vi "Tektronix ConfigOnly.vi"(5 "End Point":i32, 7 "Start Point":i32, 8 "error in (no error)":errorcluster, 9 "Waveform Width":u8(knob)=2 min=1 max=2 step=1 scale=0.0..2.0, 10 "# Average":u8(ring)=4 items=["128"=128, "64"=64, "16"=16, "4"=4], 11 "Tektronix (0::20:)":refnum<visa-resource-name>) -> (0 "error out":errorcluster, 1 "Waveform Parameters":string, 2 "Acquire Parameters":string, 3 "VISA resource name out":refnum<visa-resource-name>)   [LabVIEW 2018]
panel:
  out "concatenated string":string
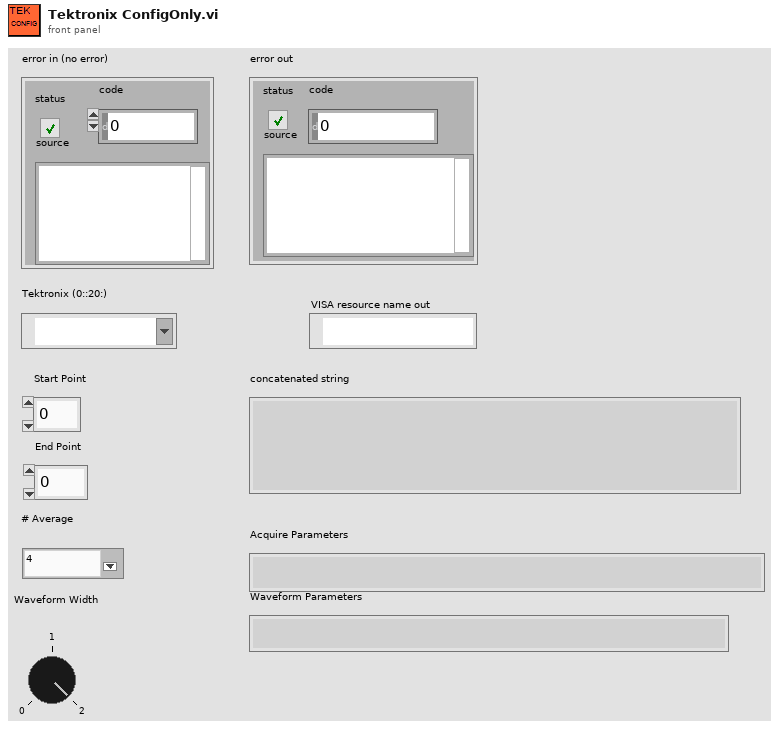
[diagram p1: front panel]
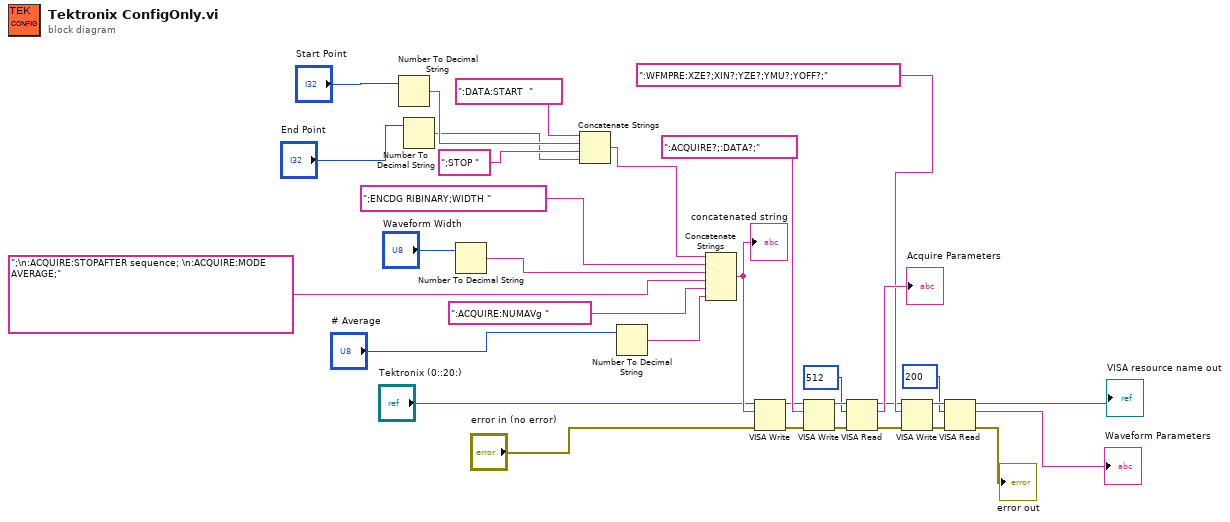
[diagram p0: block diagram]
diagram:
  n1 = Number To Decimal String(number="Start Point") -> (decimal integer string=w12:string)  [unwired: 1 in]
  n2 = Number To Decimal String(number="End Point") -> (decimal integer string=w10:string)  [unwired: 1 in]
  n3 = Number To Decimal String(number="Waveform Width") -> (decimal integer string=w1:string)  [unwired: 1 in]
  n4 = Concatenate Strings(":DATA:START  " ("string"), w12, ";STOP " ("string"), w10) -> (w4:string)
  n5 = Number To Decimal String(number="# Average") -> (decimal integer string=w17:string)  [unwired: 1 in]
  n6 = Concatenate Strings(w4, ";ENCDG RIBINARY;WIDTH " ("string"), w1, ";\n:ACQUIRE:STOPAFTER sequence; \n:ACQUIRE:MODE AVERAGE;" ("write buffer"), ":ACQUIRE:NUMAVg " ("string"), w17) -> (w19:string)
  "concatenated string" <- w19
  n7 = VISA Write(VISA resource name="Tektronix (0::20:)", write buffer=w19, error in (no error)="error in (no error)") -> (VISA resource name out=w24:refnum<visa-resource-name>, error out=w29:errorcluster)  [unwired: 1 out]
  n8 = VISA Write(VISA resource name=w24, write buffer=":ACQUIRE?;:DATA?;", error in (no error)=w29) -> (VISA resource name out=w33:refnum<visa-resource-name>, error out=w32:errorcluster)  [unwired: 1 out]
  n9 = VISA Read(VISA resource name=w33, byte count=u32 512, error in (no error)=w32) -> (VISA resource name out=w5:refnum<visa-resource-name>, read buffer=→"Acquire Parameters":string, error out=w28:errorcluster)  [unwired: 1 out]
  n10 = VISA Write(VISA resource name=w5, write buffer=":WFMPRE:XZE?;XIN?;YZE?;YMU?;YOFF?;", error in (no error)=w28) -> (VISA resource name out=w25:refnum<visa-resource-name>, error out=w27:errorcluster)  [unwired: 1 out]
  n11 = VISA Read(VISA resource name=w25, byte count=u32 200, error in (no error)=w27) -> (VISA resource name out=→"VISA resource name out":refnum<visa-resource-name>, read buffer=→"Waveform Parameters":string, error out=→"error out":errorcluster)  [unwired: 1 out]
